vi "P4CMDSub Get Working Dir.vi"(11 "files":path[](array[path])) -> (3 "working directory":path)   [LabVIEW 2017, in "NI_SCC_P4CMD.lvlib"]
uses:
  <vilib>/SourceControl/Providers/P4CMD/NI_SCC_P4CMD.lvlib
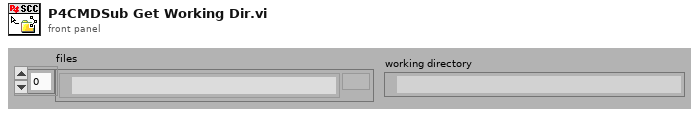
[diagram p1: front panel]
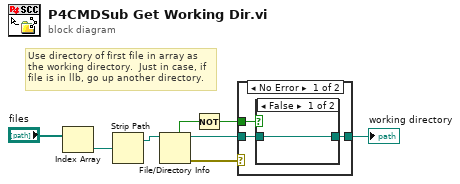
[diagram p0: block diagram]
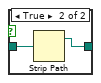
[diagram p2: hidden frame]
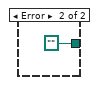
[diagram p3: hidden frame]
diagram:
  # "Use directory of first file in array as the working directory.  Just in case, if file is in llb, go up another directory."
  n1 = Index Array(array="files") -> (element=w1:path)  [unwired: 1 in]
  n2 = Strip Path(path=w1) -> (stripped path=w4:path)  [unwired: 1 out]
  n3 = File/Directory Info(path=w4) -> (path out=w6:path, directory=w5:bool, error out=w8:errorcluster)  [unwired: 1 in, 4 out]
  n4 = Not(x=w5) -> (.not. x?=w3:bool)
  n5 = case shown="No Error" w8 {
    tunnel: w3 -> [w9 _]
    tunnel: w6 -> [w11 _]
    tunnel: [w10 path ""] -> w7
    frame No Error {
      n6 = case shown="False" w9 {
        tunnel: w11 -> [w12 w14]
        tunnel: [w12 w13] -> w10
        frame False {
        }
        frame True {
          n7 = Strip Path(path=w14) -> (stripped path=w13:path)  [unwired: 1 out]
        }
      }
    }
    frame Error {
    }
  }
  "working directory" <- w7
